vi "Set_Source_ExportedVI_Data.vi"(8 "error in (no error)":errorcluster, 10 "data":T1, 11 "Class in":refnum<class "AB_Source_ExportedVI.lvclass">) -> (0 "error out":errorcluster, 3 "Class out":refnum<class "AB_Source_ExportedVI.lvclass">)   [LabVIEW 2020, in "AB_Source_ExportedVI.lvclass"]
uses:
  <vilib>/AppBuilder/AB_Classes/Source/ExportedVI/AB_Source_ExportedVI.lvclass
  <vilib>/AppBuilder/ABAPI Dist VI Proto Info New.ctl
  <vilib>/AppBuilder/AB_Classes/Source/ExportedVI/AB_Source_ExportedVI.lvclass/AB_Source_ExportedVI.ctl
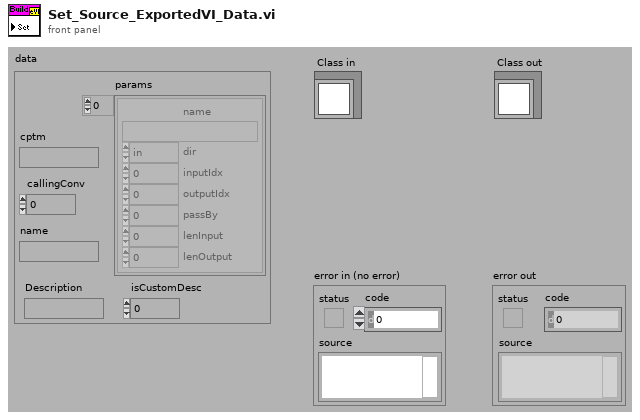
[diagram p1: front panel]
types:
  T1 = typedef "ABAPI Dist VI Proto Info New.ctl" = cluster{"cptm":string, "params":cluster{"name":string, "dir":enum32{"in", "out", "in/out", "length", "error-out"}, "inputIdx":i32, "outputIdx":i32, "passBy":i32, "lenInput":i32, "lenOutput":i32}[], "callingConv":i32, "name":string, "Description":string, "isCustomDesc":i32}
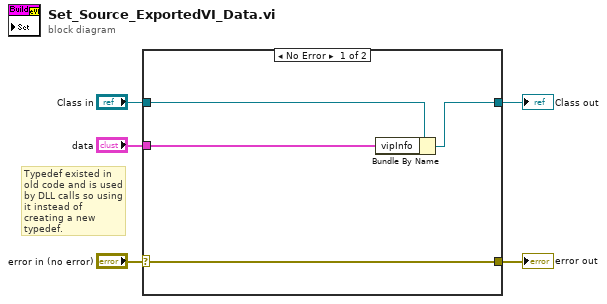
[diagram p0: block diagram]
diagram:
  # "Typedef existed in old code and is used by DLL calls so using it instead of creating a new typedef."
  n1 = case shown="No Error" "error in (no error)" {
    selector: "error in (no error)" -> [w9 w11]
    tunnel: [w9 w11] -> w4
    tunnel: "Class in" -> [w8 w10]
    tunnel: [w7 w10] -> w2
    tunnel: "data" -> [w6 _]
    frame No Error {
      n2 = Bundle By Name(cluster=w8, "vipInfo"=w6) -> (w7:refnum<class "AB_Source_ExportedVI.lvclass">)
    }
    frame Error {
    }
  }
  "error out" <- w4
  "Class out" <- w2
